vi "Autonomous Independent.vi"() -> ()   [LabVIEW 2016]
doc: "This VI is called when autonomous begins, and will automatically be terminated when autonomous ends. You can carry out timed or sensor driven robot movement independently without needing to return to the caller."
uses:
  <vilib>/Rock Robotics/WPI/Solenoid/WPI_SolenoidValue.ctl
  <vilib>/Rock Robotics/WPI/Utilities/WPI_GetSetVariantRefNum.vi
  <vilib>/Rock Robotics/Network Tables/NT Write Numeric Array.vi
  <vilib>/Rock Robotics/Network Tables/NT Read String.vi
  <vilib>/Rock Robotics/WPI/Solenoid/WPI_SolenoidSetEnum.vi
  Robot Global Data.vi
  <vilib>/Rock Robotics/Network Tables/NT Read Number.vi
panel:
  out "center x 8":dbl
  out "center y 8":dbl
  out "turn speed 7":dbl
  out "left motor 7":dbl
  out "right motor 7":dbl
  out "center x 7":dbl
  out "center y 7":dbl
  out "turn speed 6":dbl
  out "left motor 6":dbl
  out "right motor 6":dbl
  out "center x 6":dbl
  out "center y 6":dbl
  out "turn speed 5":dbl
  out "left motor 5":dbl
  out "right motor 5":dbl
  out "center x 2":dbl
  out "center y 2":dbl
  out "turn speed":dbl
  in  "turn offset":dbl
  out "left motor":dbl
  out "right motor":dbl
  in  "turn gain":dbl
  in  "drive gain":dbl
  in  "max drive speed":dbl
  in  "min drive speed":dbl
  in  "stop distance":dbl
  out "center x":dbl
  out "center y":dbl
  out "motor speed":dbl
  in  "setpoint":dbl
  # "Be sure to right-click and choose Data Operations>>Make Current Value default if you want to save the array values with the VI"
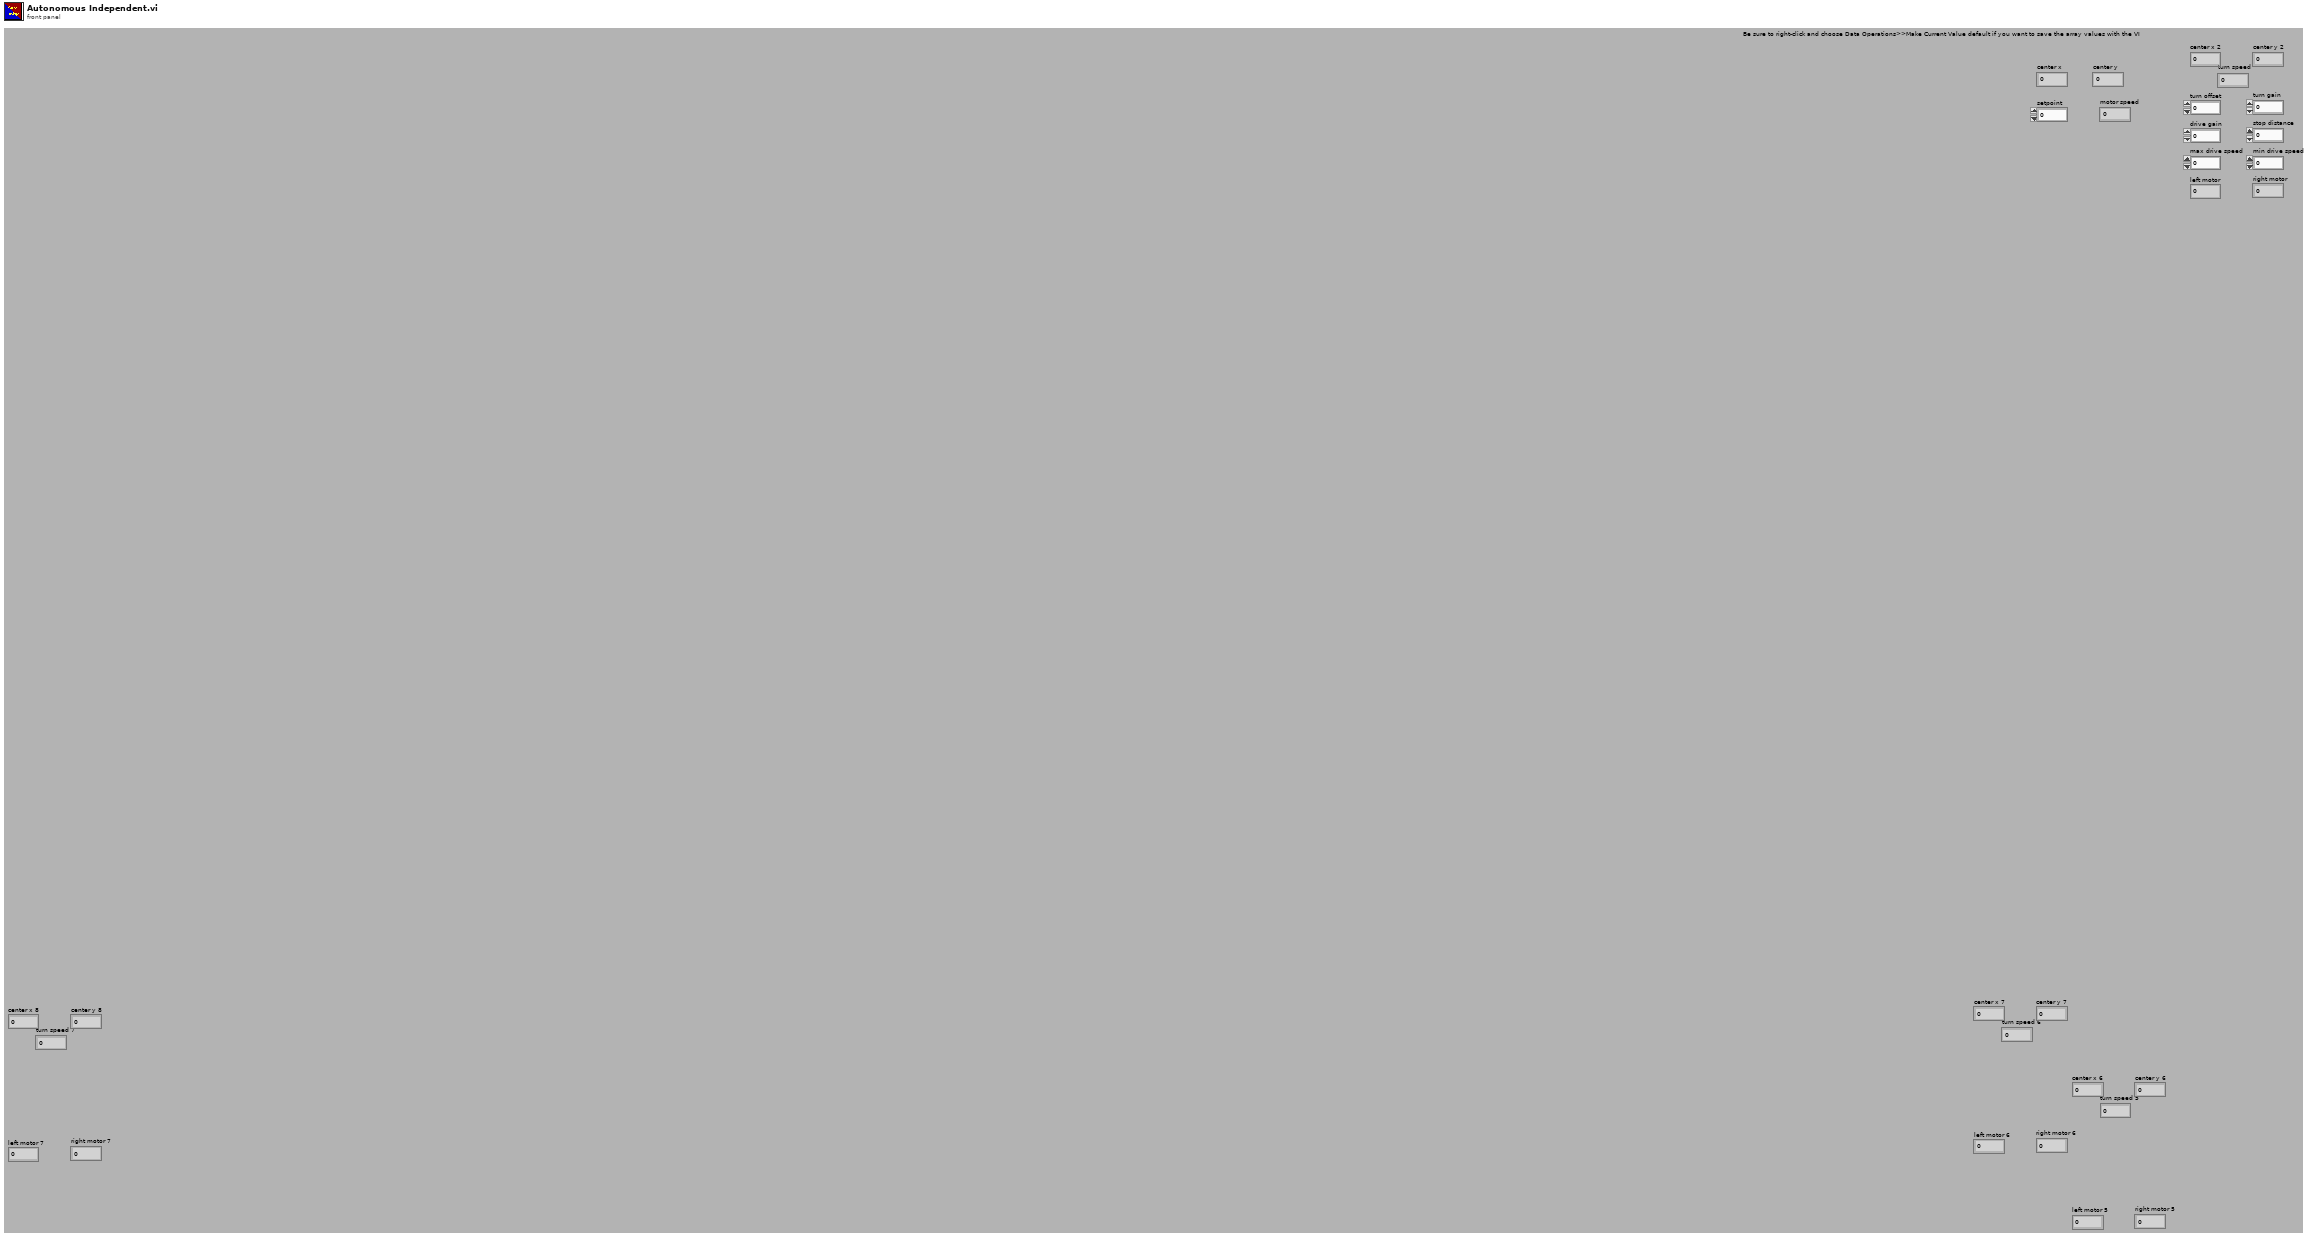
[diagram p1: front panel]
types:
  T1 = cluster{"Distance (ft)":dbl, "Score":dbl, "Normalized":cluster{"Center":cluster{dbl, dbl}, "Rectangle":cluster{"Numeric":dbl, "Numeric 2":dbl, "Numeric 3":dbl, "Numeric 5":dbl}}, "Pixels":cluster{"Center":cluster{dbl, dbl}, "Rectangle":cluster{"Numeric":dbl, "Numeric 2":dbl, "Numeric 3":dbl, "Numeric 5":dbl}}}
  T2 = typedef "WPI_RobotDriveDevRef.ctl" = cluster{"DevStatus":errorcluster, "Motors[]":T3[], "Square Inputs":bool, "Max Output":dbl}
  T3 = typedef "WPI_MotorControlDeviceRef.ctl" = cluster{"DeviceStatus":errorcluster, "Type":T4, "PWM":cluster{"PWM Channel":T5, "DeadBand":T6}, "CAN":cluster{"Device Number":u8, "SetOutput VI Ref":variant, "GetOutput VI Ref":variant, "Enable VI Ref":variant, "Disable VI Ref":variant, "Data":variant}, "Invert":bool}
  T4 = typedef "WPI_MotorControlType.ctl" = enum16{"PWM", "CAN"}
  T5 = typedef "FPGA_DIOPWMChannel.ctl" = enum8{"PWM 0", "PWM 1", "PWM 2", "PWM 3", "PWM 4", "PWM 5", "PWM 6", "PWM 7", "PWM 8", "PWM 9", "PWM MXP 0", "PWM MXP 1", "PWM MXP 2", "PWM MXP 3", "PWM MXP 4", "PWM MXP 5", "PWM MXP 6", "PWM MXP 7", "PWM MXP 8", "PWM MXP 9", "Invalid"}
  T6 = typedef "WPI_PWMDeadband.ctl" = cluster{"Name":string, "maxPositivePwm":i32, "minPositivePwm":i32, "centerPwm":i32, "maxNegativePwm":i32, "minNegativePwm":i32, "angularRange":u16}
  T7 = typedef "WPI_JoystickDevRef.ctl" = cluster{"Device":T8}
  T8 = typedef "WPI_JoystickDeviceEnum.ctl" = enum16{"USB 0", "USB 1", "USB 2", "USB 3", "USB 4", "USB 5"}
  T9 = typedef "WPI_SolenoidValue.ctl" = enum16{"Off", "On", "Forward", "Reverse"}
  T10 = typedef "WPI_EncoderDevRef.ctl" = cluster{"DevStatus":errorcluster, "EncoderIndex":T11, "CounterIndex":T12, "DistancePerCount":dbl, "Decoding Type":T13}
  T11 = typedef "FPGA_EncoderIdx.ctl" = enum8{"Enc 0", "Enc 1", "Enc 2", "Enc 3", "Enc 4", "Enc 5", "Enc 6", "Enc 7", "Invalid"}
  T12 = typedef "FPGA_CounterCtrSystemIndex.ctl" = enum8{"Ctr 0", "Ctr 1", "Ctr 2", "Ctr 3", "Ctr 4", "Ctr 5", "Ctr 6", "Ctr 7", "Invalid"}
  T13 = typedef "WPI_EncoderType.ctl" = enum16{"1x", "2x", "4x"}
  T14 = typedef "WPI_SolenoidDevRef.ctl" = cluster{"DevStatus":errorcluster, "Pneumatics Control Module":u8, "Forward Solenoid Channel":T15, "Reverse Solenoid Channel":T15}
  T15 = typedef "WPI_SolenoidChannel.ctl" = enum8{"Solenoid 0", "Solenoid 1", "Solenoid 2", "Solenoid 3", "Solenoid 4", "Solenoid 5", "Solenoid 6", "Solenoid 7", "Invalid"}
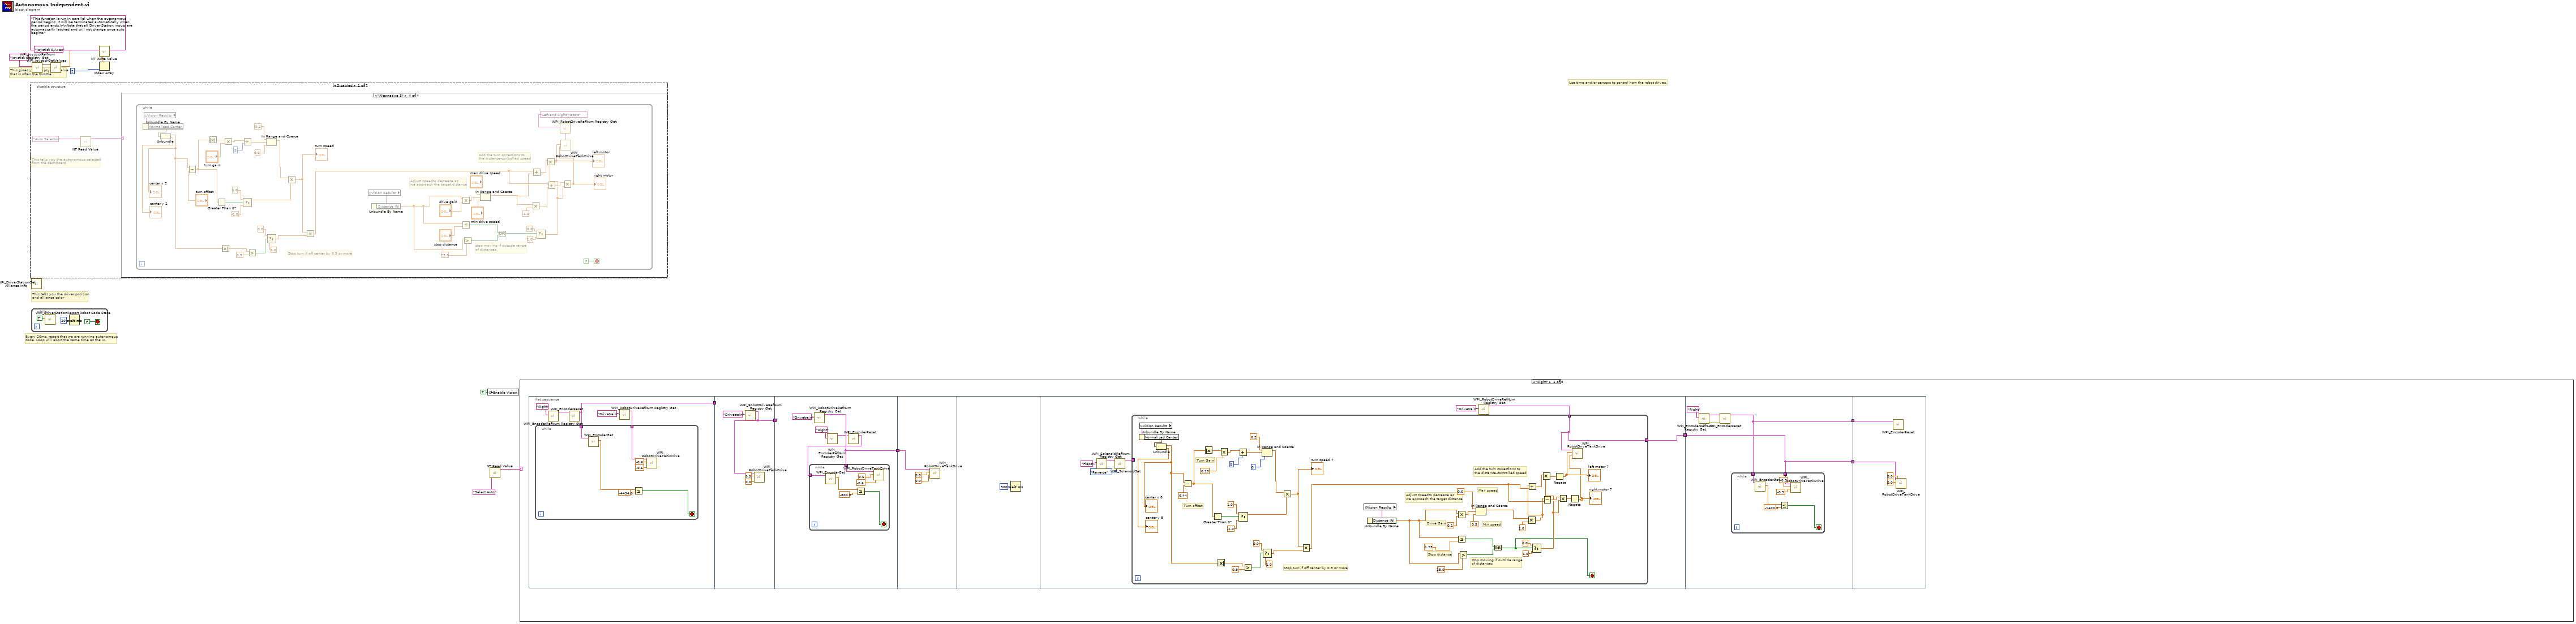
[diagram p0: block diagram]
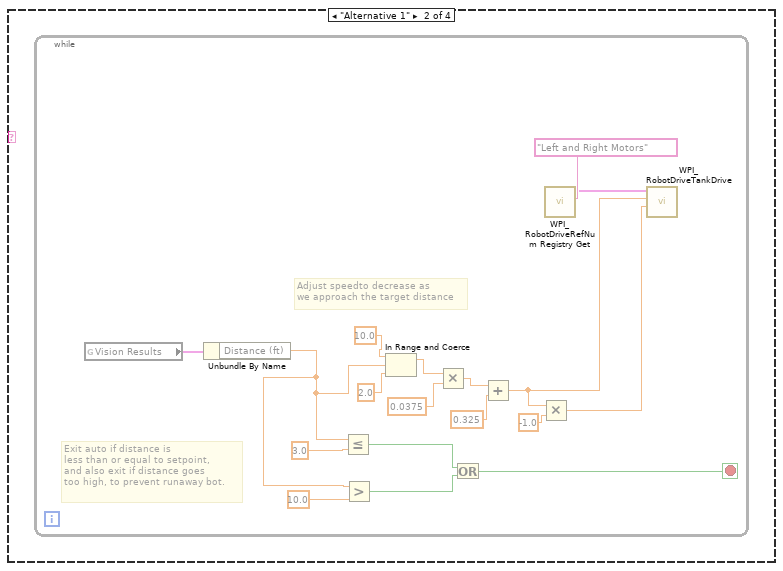
[diagram p3: hidden frame]
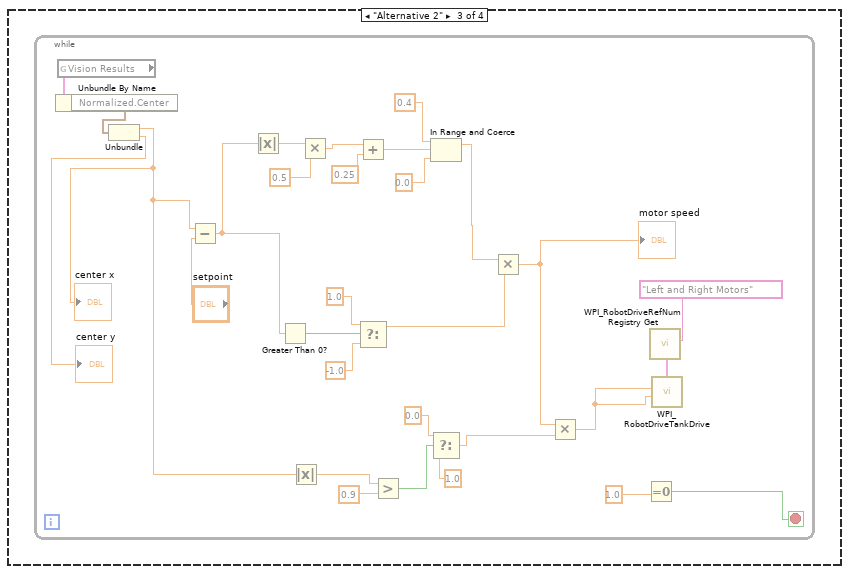
[diagram p4: hidden frame]
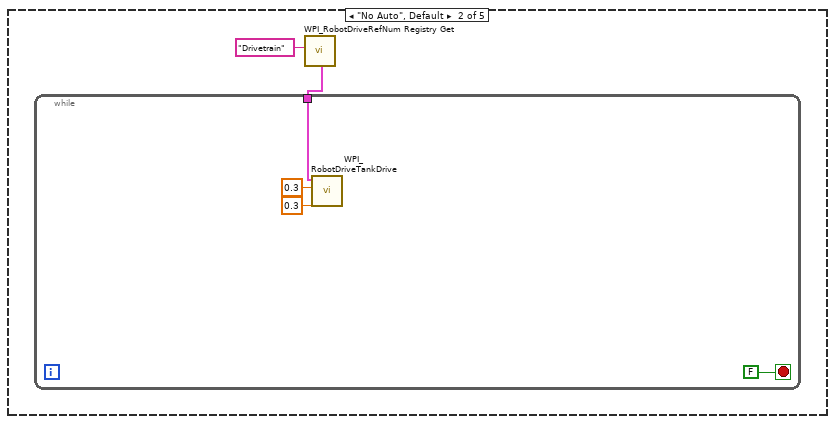
[diagram p6: hidden frame]
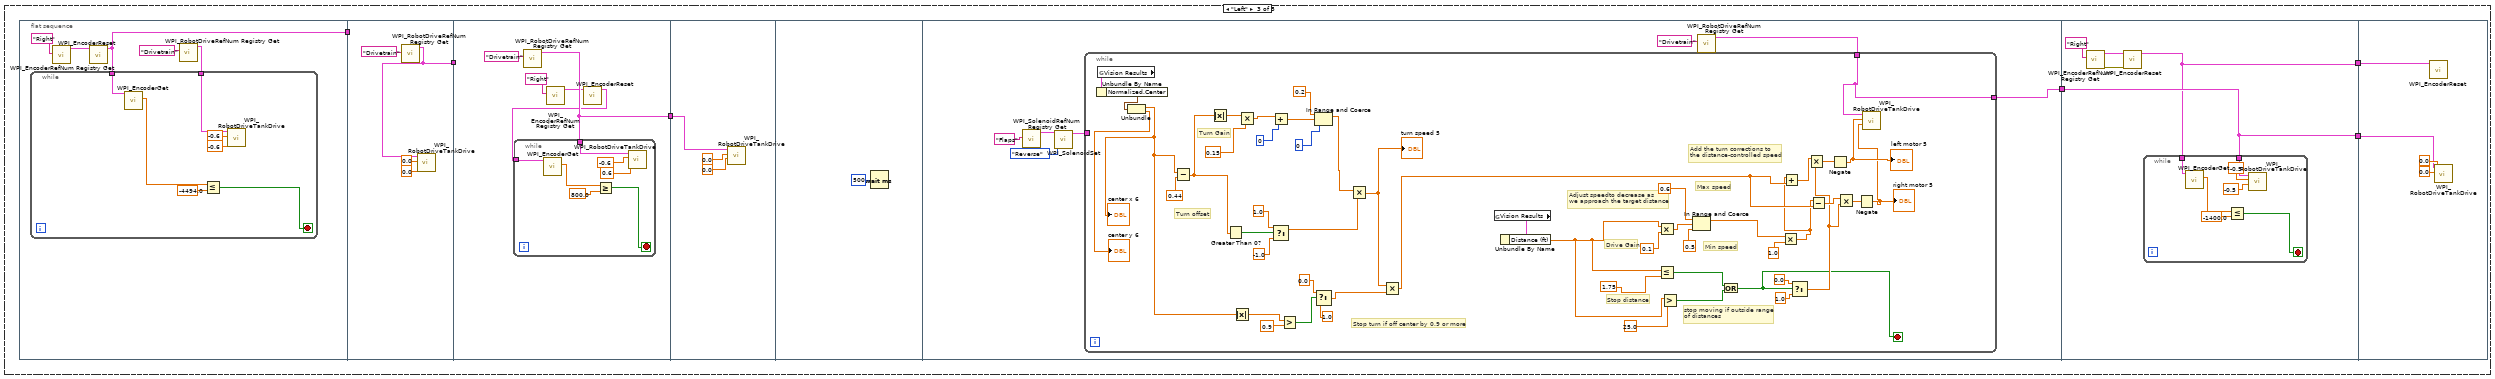
[diagram p7: hidden frame]
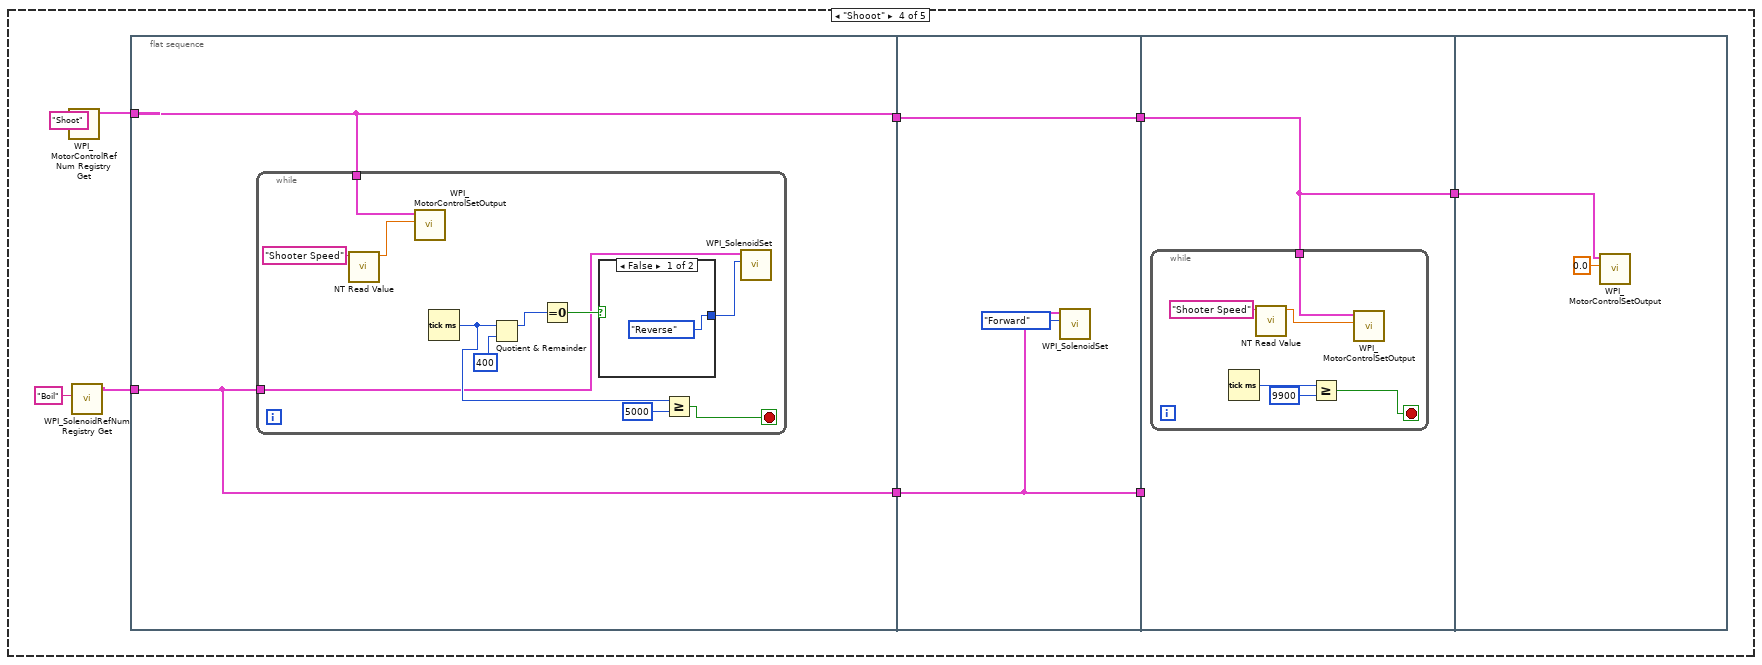
[diagram p8: hidden frame]
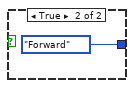
[diagram p9: hidden frame]
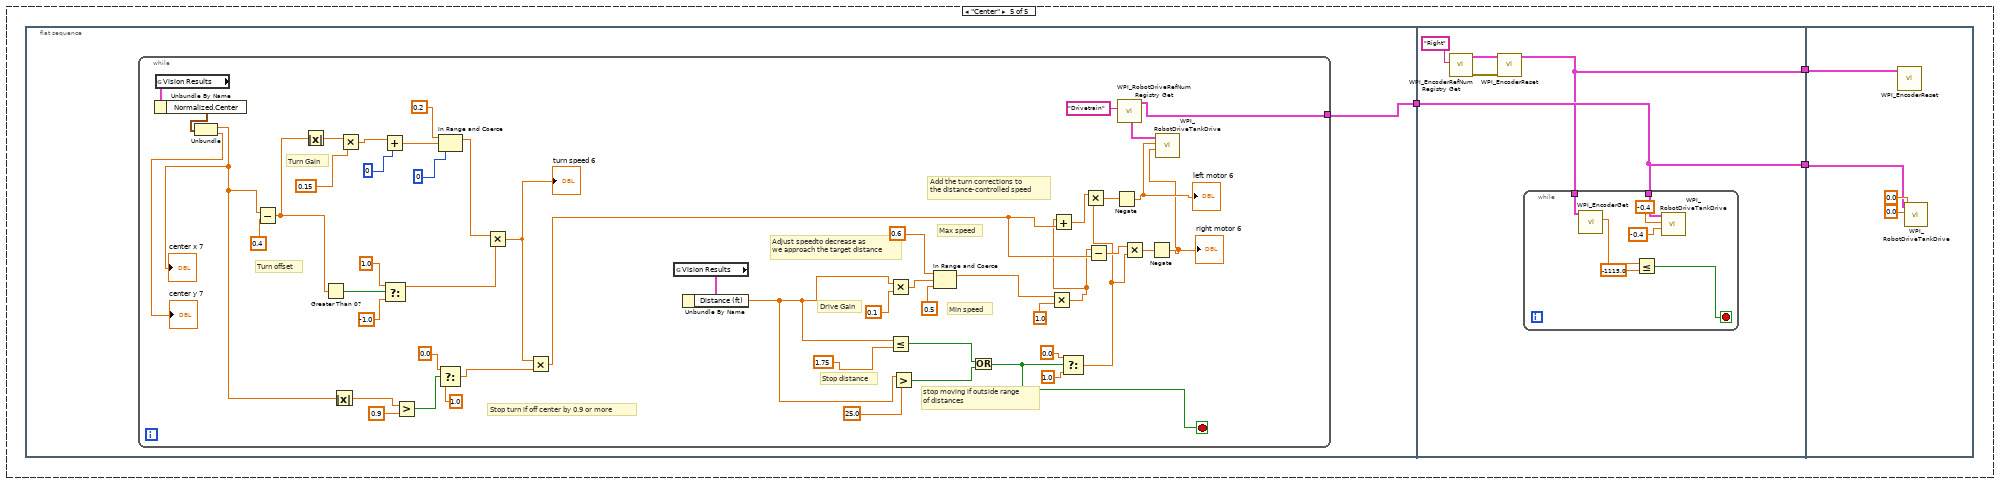
[diagram p10: hidden frame]
diagram:
  (unwired) "This function is run in parallel when the autonomous period begins. It will be terminated automatically when the period ends.\n\nNote that all Driver Station inputs are automatically latched and will not change once auto begins."
  # "Every 20ms, report that we are running autonomous\ncode. Loop will abort the same time as the VI."
  # "This gives you the joystick value\nthat is often the throttle"
  # "Use time and/or sensors to control how the robot drives."
  # "This tells you the driver position\nand alliance color"
  n1 = disable-structure shown="Disabled" {
    frame Disabled {
      # "This tells you the autonomous selected\nfrom the dashboard"
      n2 = call-poly <vilib>:"NT Read Value.vi"("Name"="Auto Selector") -> ("String"=w9:string)  [unwired: 9 in, 1 out]
      n3 = case shown="\"Alternative 3\"" w9 {
        frame Default {
          # "You can put your main auto here, or you can right-click on the case and make any\nother frame be the default case."
          # "This is the frame that will execute if no selection is made, or if it is not recognized"
        }
        frame "Alternative 1" {
          n4 = while {
            stop <- w11 stop-if-true
            # "Adjust speedto decrease as \nwe approach the target distance"
            # "Exit auto if distance is\nless than or equal to setpoint,\nand also exit if distance goes \ntoo high, to prevent runaway bot."
            n5 = global read "Robot Global Data.vi" "Vision Results"() -> (w28:T1)
            n6 = Unbundle By Name(w28) -> ("Distance (ft)"=w15:dbl)
            n7 = Less Or Equal?(x=w15, y=3.0) -> (x <= y?=w13:bool)
            n8 = Greater?(x=w15, y=10.0) -> (0:w12:bool)
            n9 = In Range and Coerce(upper limit=10.0 ("y"), x=w15, lower limit=2.0 ("y")) -> (coerced(x)=w22:dbl)  [unwired: 1 out]
            n10 = Multiply(x=w22, y=0.0375) -> (x*y=w20:dbl)
            n11 = Or(x=w13, y=w12) -> (x .or. y?=w11:bool)
            n12 = Add(x=w20, y=0.325) -> (x+y=w18:dbl)
            n13 = Multiply(x=w18, y=-1.0) -> (x*y=w16:dbl)
            n14 = call <vilib>:"WPI_RobotDriveRefNum Registry Get.vi"("refnum name"="Left and Right Motors") -> ("RobotDriveDevRef"=w26:T2)  [unwired: 9 in, 1 out]
            n15 = call <vilib>:"WPI_RobotDriveTankDrive.vi"("Right axis value"=w16, "Left axis value"=w18, "RobotDriveDevRef"=w26) -> ()  [unwired: 6 in, 3 out]
          }
        }
        frame "Alternative 2" {
          n16 = while {
            stop <- w32 stop-if-true
            n17 = global read "Robot Global Data.vi" "Vision Results"() -> (w58:T1)
            n18 = Unbundle By Name(w58) -> ("Normalized.Center"=w54:cluster{dbl, dbl})
            n19 = Unbundle(w54) -> (w30:dbl, →"center y":dbl)
            "center x" <- w30
            n20 = Subtract(x=w30, y="setpoint") -> (x-y=w29:dbl)
            n21 = Absolute Value(x=w29) -> (abs(x)=w46:dbl)
            n22 = Greater Than 0?(x=w29) -> (x > 0?=w51:bool)
            n23 = Absolute Value(x=w30) -> (abs(x)=w53:dbl)
            n24 = Multiply(x=w46, y=0.5) -> (x*y=w44:dbl)
            n25 = Add(x=w44, y=0.25) -> (x+y=w42:dbl)
            n26 = Select(t=1.0, s=w51, f=-1.0 ("t")) -> (s? t:f=w48:dbl)
            n27 = Greater?(x=w53, y=0.9) -> (0:w39:bool)
            n28 = In Range and Coerce(upper limit=0.4, x=w42, lower limit=0.0) -> (coerced(x)=w40:dbl)  [unwired: 1 out]
            n29 = Select(t=0.0, s=w39, f=1.0 ("t")) -> (s? t:f=w36:dbl)
            n30 = Multiply(x=w40, y=w48) -> (x*y=w35:dbl)
            "motor speed" <- w35
            n31 = Multiply(x=w35, y=w36) -> (x*y=w34:dbl)
            n32 = Equal To 0?(x=1.0 ("t")) -> (x = 0?=w32:bool)
            n33 = call <vilib>:"WPI_RobotDriveRefNum Registry Get.vi"("refnum name"="Left and Right Motors") -> ("RobotDriveDevRef"=w55:T2)  [unwired: 9 in, 1 out]
            n34 = call <vilib>:"WPI_RobotDriveTankDrive.vi"("Right axis value"=w34, "Left axis value"=w34, "RobotDriveDevRef"=w55) -> ()  [unwired: 6 in, 3 out]
          }
        }
        frame "Alternative 3" {
          n35 = while {
            stop <- FALSE stop-if-true
            # "stop moving if outside range\nof distances"
            # "Stop turn if off center by 0.9 or more"
            # "Add the turn corrections to \nthe distance-controlled speed"
            # "Adjust speedto decrease as \nwe approach the target distance"
            n36 = global read "Robot Global Data.vi" "Vision Results"() -> (w108:T1)
            n37 = Unbundle By Name(w108) -> ("Normalized.Center"=w106:cluster{dbl, dbl})
            n38 = Unbundle(w106) -> (w86:dbl, →"center y 2":dbl)
            "center x 2" <- w86
            n39 = Subtract(x=w86, y="turn offset") -> (x-y=w85:dbl)
            n40 = Absolute Value(x=w85) -> (abs(x)=w98:dbl)
            n41 = Greater Than 0?(x=w85) -> (x > 0?=w103:bool)
            n42 = Absolute Value(x=w86) -> (abs(x)=w105:dbl)
            n43 = Multiply(x=w98, y="turn gain") -> (x*y=w97:dbl)
            n44 = Add(x=w97, y=0) -> (x+y=w95:dbl)
            n45 = Select(t=1.0, s=w103, f=-1.0 ("t")) -> (s? t:f=w100:dbl)
            n46 = Greater?(x=w105, y=0.9) -> (0:w92:bool)
            n47 = In Range and Coerce(upper limit=0.2, x=w95, lower limit=0.0) -> (coerced(x)=w93:dbl)  [unwired: 1 out]
            n48 = Select(t=0.0, s=w92, f=1.0 ("t")) -> (s? t:f=w89:dbl)
            n49 = Multiply(x=w93, y=w100) -> (x*y=w88:dbl)
            "turn speed" <- w88
            n50 = Multiply(x=w88, y=w89) -> (x*y=w77:dbl)
            n51 = global read "Robot Global Data.vi" "Vision Results"() -> (w84:T1)
            n52 = Unbundle By Name(w84) -> ("Distance (ft)"=w65:dbl)
            n53 = Multiply(x=w65, y="drive gain") -> (x*y=w64:dbl)
            n54 = Less Or Equal?(x=w65, y="stop distance") -> (x <= y?=w79:bool)
            n55 = Greater?(x=w65, y=25.0) -> (0:w78:bool)
            n56 = In Range and Coerce(upper limit="max drive speed", x=w64, lower limit="min drive speed") -> (coerced(x)=w61:dbl)  [unwired: 1 out]
            n57 = Or(x=w79, y=w78) -> (x .or. y?=w75:bool)
            n58 = Multiply(x=w61, y=-1.0) -> (x*y=w76:dbl)
            n59 = Add(x=w77, y=w61) -> (x+y=w72:dbl)
            n60 = Select(t=0.0, s=w75, f=1.0 ("t")) -> (s? t:f=w70:dbl)
            n61 = Multiply(x=w72, y=w70) -> (x*y=w69:dbl)
            "left motor" <- w69
            n62 = Add(x=w77, y=w76) -> (x+y=w71:dbl)
            n63 = call <vilib>:"WPI_RobotDriveRefNum Registry Get.vi"("refnum name"="Left and Right Motors") -> ("RobotDriveDevRef"=w82:T2)  [unwired: 9 in, 1 out]
            n64 = Multiply(x=w71, y=w70) -> (x*y=w68:dbl)
            "right motor" <- w68
            n65 = call <vilib>:"WPI_RobotDriveTankDrive.vi"("Right axis value"=w68, "Left axis value"=w69, "RobotDriveDevRef"=w82) -> ()  [unwired: 6 in, 3 out]
          }
        }
      }
    }
    frame Enabled {
    }
  }
  n66 = while {
    stop <- FALSE stop-if-true
    n67 = call <vilib>:"WPI_DriverStationReport Robot Code State.vi"("Autonomous"=TRUE) -> ()  [unwired: 10 in, 1 out]
    n68 = Wait (ms)(milliseconds to wait=u32 20) -> ()  [unwired: 1 out]
  }
  n69 = call <vilib>:"WPI_DriverStationGet Alliance Info.vi"() -> ()  [unwired: 12 out]
  n70 = call <vilib>:"WPI_JoystickRefNum Registry Get.vi"("refnum name"="Joystick 0") -> ("JoystickDevRef"=w7:T7)  [unwired: 1 in, 9 out]
  n71 = call <vilib>:"WPI_JoystickGetValues.vi"("JoystickDevRef"=w7) -> ("Axes"=w5:dbl[])  [unwired: 6 in, 4 out]
  n72 = call-poly <vilib>:"NT Write Value.vi"("Numeric Array"=w5, "Name"="Joystick 0/Axes") -> ()  [unwired: 9 in, 1 out]
  n73 = Index Array(array=w5, index=2) -> ()  [unwired: 1 out]
  n74 = global write "Robot Global Data.vi" "Enable Vision"(TRUE ("Enable Vision")) -> ()
  n75 = call-poly <vilib>:"NT Read Value.vi"("Name"="Select Auto") -> ("String"=w2:string)  [unwired: 9 in, 1 out]
  n76 = case shown="\"Right\"" w2 {
    frame "Right" {
      n77 = flat-sequence {
        tunnel: [w118] -> w117
        tunnel: [w130] -> w116
        tunnel: w117 -> [_]
        tunnel: w116 -> [_]
        tunnel: [w137] -> w115
        tunnel: w115 -> [w146]
        tunnel: [w156] -> w114
        tunnel: w114 -> [w208]
        tunnel: [w208] -> w113
        tunnel: [w207] -> w112
        tunnel: w113 -> [w220]
        tunnel: w112 -> [w219]
        frame #0 {
          n78 = call <vilib>:"WPI_EncoderRefNum Registry Get.vi"("refnum name"="Right") -> ("EncoderDevRef"=w122:T10)  [unwired: 9 in, 1 out]
          n79 = call <vilib>:"WPI_EncoderReset.vi"("EncoderDevRef"=w122) -> ("EncoderDevRef"=w118:T10)  [unwired: 9 in, 1 out]
          n80 = call <vilib>:"WPI_RobotDriveRefNum Registry Get.vi"("refnum name"="Drivetrain") -> ("RobotDriveDevRef"=w119:T2)  [unwired: 9 in, 1 out]
          n81 = while {
            tunnel: w118 -> [w126]
            tunnel: w119 -> [w125]
            stop <- w127 stop-if-true
            n82 = call <vilib>:"WPI_EncoderGet.vi"("EncoderDevRef"=w126) -> ("Distance"=w129:dbl)  [unwired: 5 in, 5 out]
            n83 = Less Or Equal?(x=w129, y=-4494.0) -> (x <= y?=w127:bool)
            n84 = call <vilib>:"WPI_RobotDriveTankDrive.vi"("Right axis value"=-0.6, "Left axis value"=-0.6, "RobotDriveDevRef"=w125) -> ()  [unwired: 6 in, 3 out]
          }
        }
        frame #1 {
          n85 = call <vilib>:"WPI_RobotDriveRefNum Registry Get.vi"("refnum name"="Drivetrain") -> ("RobotDriveDevRef"=w130:T2)  [unwired: 9 in, 1 out]
          n86 = call <vilib>:"WPI_RobotDriveTankDrive.vi"("Right axis value"=0.0, "Left axis value"=0.0, "RobotDriveDevRef"=w130) -> ()  [unwired: 6 in, 3 out]
        }
        frame #2 {
          n87 = call <vilib>:"WPI_RobotDriveRefNum Registry Get.vi"("refnum name"="Drivetrain") -> ("RobotDriveDevRef"=w137:T2)  [unwired: 9 in, 1 out]
          n88 = call <vilib>:"WPI_EncoderRefNum Registry Get.vi"("refnum name"="Right") -> ("EncoderDevRef"=w136:T10)  [unwired: 9 in, 1 out]
          n89 = call <vilib>:"WPI_EncoderReset.vi"("EncoderDevRef"=w136) -> ("EncoderDevRef"=w134:T10)  [unwired: 9 in, 1 out]
          n90 = while {
            tunnel: w137 -> [w142]
            tunnel: w134 -> [w141]
            stop <- w145 stop-if-true
            n91 = call <vilib>:"WPI_EncoderGet.vi"("EncoderDevRef"=w141) -> ("Distance"=w140:dbl)  [unwired: 5 in, 5 out]
            n92 = Less Or Equal?(x=w140, y=-800.0) -> (x <= y?=w145:bool)
            n93 = call <vilib>:"WPI_RobotDriveTankDrive.vi"("Right axis value"=-0.6, "Left axis value"=0.6, "RobotDriveDevRef"=w142) -> ()  [unwired: 6 in, 3 out]
          }
        }
        frame #3 {
          n94 = call <vilib>:"WPI_RobotDriveTankDrive.vi"("Right axis value"=0.0, "Left axis value"=0.0, "RobotDriveDevRef"=w146) -> ()  [unwired: 6 in, 3 out]
        }
        frame #4 {
          n95 = Wait (ms)(milliseconds to wait=u32 500) -> ()  [unwired: 1 out]
        }
        frame #5 {
          n96 = call <vilib>:"WPI_SolenoidRefNum Registry Get.vi"("refnum name"="Flaps") -> ("SolenoidDevRef"=w154:T14)  [unwired: 9 in, 1 out]
          n97 = call-poly <vilib>:"WPI_SolenoidSet.vi"("Value"=WPI_SolenoidValue."Reverse", "SolenoidDevRef"=w154) -> ("SolenoidDevRef"=w150:T14)  [unwired: 8 in, 1 out]
          n98 = call <vilib>:"WPI_RobotDriveRefNum Registry Get.vi"("refnum name"="Drivetrain") -> ("RobotDriveDevRef"=w151:T2)  [unwired: 9 in, 1 out]
          n99 = while {
            tunnel: [w158] -> w156
            tunnel: w151 -> [w158]
            tunnel: w150 -> [_]
            stop <- w157 stop-if-true
            # "Min speed"
            # "Max speed"
            # "Stop distance"
            # "Drive Gain"
            # "Turn offset"
            # "Turn Gain"
            # "stop moving if outside range\nof distances"
            # "Stop turn if off center by 0.9 or more"
            # "Add the turn corrections to \nthe distance-controlled speed"
            # "Adjust speedto decrease as \nwe approach the target distance"
            n100 = global read "Robot Global Data.vi" "Vision Results"() -> (w206:T1)
            n101 = Unbundle By Name(w206) -> ("Normalized.Center"=w204:cluster{dbl, dbl})
            n102 = Unbundle(w204) -> (w185:dbl, →"center y 8":dbl)
            "center x 8" <- w185
            n103 = Subtract(x=w185, y=0.44) -> (x-y=w184:dbl)
            n104 = Absolute Value(x=w184) -> (abs(x)=w196:dbl)
            n105 = Greater Than 0?(x=w184) -> (x > 0?=w201:bool)
            n106 = Absolute Value(x=w185) -> (abs(x)=w203:dbl)
            n107 = Multiply(x=w196, y=0.15) -> (x*y=w195:dbl)
            n108 = Add(x=w195, y=0) -> (x+y=w193:dbl)
            n109 = Select(t=1.0, s=w201, f=-1.0 ("t")) -> (s? t:f=w198:dbl)
            n110 = Greater?(x=w203, y=0.9) -> (0:w190:bool)
            n111 = In Range and Coerce(upper limit=0.2, x=w193, lower limit=0) -> (coerced(x)=w191:dbl)  [unwired: 1 out]
            n112 = Select(t=0.0, s=w190, f=1.0 ("t")) -> (s? t:f=w187:dbl)
            n113 = Multiply(x=w191, y=w198) -> (x*y=w186:dbl)
            "turn speed 7" <- w186
            n114 = Multiply(x=w186, y=w187) -> (x*y=w164:dbl)
            n115 = global read "Robot Global Data.vi" "Vision Results"() -> (w183:T1)
            n116 = Unbundle By Name(w183) -> ("Distance (ft)"=w173:dbl)
            n117 = Multiply(x=w173, y=0.1) -> (x*y=w172:dbl)
            n118 = Less Or Equal?(x=w173, y=1.75) -> (x <= y?=w180:bool)
            n119 = Greater?(x=w173, y=25.0) -> (0:w179:bool)
            n120 = In Range and Coerce(upper limit=0.6, x=w172, lower limit=0.5) -> (coerced(x)=w171:dbl)  [unwired: 1 out]
            n121 = Or(x=w180, y=w179) -> (x .or. y?=w157:bool)
            n122 = Multiply(x=w171, y=1.0) -> (x*y=w163:dbl)
            n123 = Add(x=w163, y=w164) -> (x+y=w176:dbl)
            n124 = Select(t=0.0, s=w157, f=1.0 ("t")) -> (s? t:f=w174:dbl)
            n125 = Multiply(x=w176, y=w174) -> (x*y=w162:dbl)
            n126 = Subtract(x=w163, y=w164) -> (x-y=w175:dbl)
            n127 = Negate(x=w162) -> (-x=w161:dbl)
            "left motor 7" <- w161
            n128 = Multiply(x=w175, y=w174) -> (x*y=w160:dbl)
            n129 = Negate(x=w160) -> (-x=w159:dbl)
            "right motor 7" <- w159
            n130 = call <vilib>:"WPI_RobotDriveTankDrive.vi"("Right axis value"=w159, "Left axis value"=w161, "RobotDriveDevRef"=w158) -> ()  [unwired: 6 in, 3 out]
          }
        }
        frame #6 {
          n131 = call <vilib>:"WPI_EncoderRefNum Registry Get.vi"("refnum name"="Right") -> ("error out"=w210:errorcluster, "EncoderDevRef"=w209:T10)  [unwired: 9 in]
          n132 = call <vilib>:"WPI_EncoderReset.vi"("error in (no error)"=w210, "EncoderDevRef"=w209) -> ("EncoderDevRef"=w207:T10)  [unwired: 8 in, 1 out]
          n133 = while {
            tunnel: w207 -> [w218]
            tunnel: w208 -> [w214]
            stop <- w215 stop-if-true
            n134 = call <vilib>:"WPI_EncoderGet.vi"("EncoderDevRef"=w218) -> ("Distance"=w217:dbl)  [unwired: 5 in, 5 out]
            n135 = Less Or Equal?(x=w217, y=-1400.0) -> (x <= y?=w215:bool)
            n136 = call <vilib>:"WPI_RobotDriveTankDrive.vi"("Right axis value"=-0.5 ("Left axis value"), "Left axis value"=-0.5 ("Right axis value"), "RobotDriveDevRef"=w214) -> ()  [unwired: 6 in, 3 out]
          }
        }
        frame #7 {
          n137 = call <vilib>:"WPI_EncoderReset.vi"("EncoderDevRef"=w219) -> ()  [unwired: 9 in, 2 out]
          n138 = call <vilib>:"WPI_RobotDriveTankDrive.vi"("Right axis value"=0.0, "Left axis value"=0.0, "RobotDriveDevRef"=w220) -> ()  [unwired: 6 in, 3 out]
        }
      }
    }
    frame "No Auto", Default {
      n139 = call <vilib>:"WPI_RobotDriveRefNum Registry Get.vi"("refnum name"="Drivetrain") -> ("RobotDriveDevRef"=w223:T2)  [unwired: 9 in, 1 out]
      n140 = while {
        tunnel: w223 -> [w225]
        stop <- FALSE stop-if-true
        n141 = call <vilib>:"WPI_RobotDriveTankDrive.vi"("Right axis value"=0.3, "Left axis value"=0.3, "RobotDriveDevRef"=w225) -> ()  [unwired: 6 in, 3 out]
      }
    }
    frame "Left" {
      n142 = flat-sequence {
        tunnel: [w235] -> w229
        tunnel: [w247] -> w230
        tunnel: w229 -> [_]
        tunnel: w230 -> [_]
        tunnel: [w254] -> w231
        tunnel: w231 -> [w263]
        tunnel: [w273] -> w234
        tunnel: w234 -> [w325]
        tunnel: [w325] -> w233
        tunnel: [w324] -> w232
        tunnel: w233 -> [w337]
        tunnel: w232 -> [w336]
        frame #0 {
          n143 = call <vilib>:"WPI_EncoderRefNum Registry Get.vi"("refnum name"="Right") -> ("EncoderDevRef"=w239:T10)  [unwired: 9 in, 1 out]
          n144 = call <vilib>:"WPI_EncoderReset.vi"("EncoderDevRef"=w239) -> ("EncoderDevRef"=w235:T10)  [unwired: 9 in, 1 out]
          n145 = call <vilib>:"WPI_RobotDriveRefNum Registry Get.vi"("refnum name"="Drivetrain") -> ("RobotDriveDevRef"=w236:T2)  [unwired: 9 in, 1 out]
          n146 = while {
            tunnel: w235 -> [w243]
            tunnel: w236 -> [w242]
            stop <- w244 stop-if-true
            n147 = call <vilib>:"WPI_EncoderGet.vi"("EncoderDevRef"=w243) -> ("Distance"=w246:dbl)  [unwired: 5 in, 5 out]
            n148 = Less Or Equal?(x=w246, y=-4494.0) -> (x <= y?=w244:bool)
            n149 = call <vilib>:"WPI_RobotDriveTankDrive.vi"("Right axis value"=-0.6, "Left axis value"=-0.6, "RobotDriveDevRef"=w242) -> ()  [unwired: 6 in, 3 out]
          }
        }
        frame #1 {
          n150 = call <vilib>:"WPI_RobotDriveRefNum Registry Get.vi"("refnum name"="Drivetrain") -> ("RobotDriveDevRef"=w247:T2)  [unwired: 9 in, 1 out]
          n151 = call <vilib>:"WPI_RobotDriveTankDrive.vi"("Right axis value"=0.0, "Left axis value"=0.0, "RobotDriveDevRef"=w247) -> ()  [unwired: 6 in, 3 out]
        }
        frame #2 {
          n152 = call <vilib>:"WPI_RobotDriveRefNum Registry Get.vi"("refnum name"="Drivetrain") -> ("RobotDriveDevRef"=w254:T2)  [unwired: 9 in, 1 out]
          n153 = call <vilib>:"WPI_EncoderRefNum Registry Get.vi"("refnum name"="Right") -> ("EncoderDevRef"=w253:T10)  [unwired: 9 in, 1 out]
          n154 = call <vilib>:"WPI_EncoderReset.vi"("EncoderDevRef"=w253) -> ("EncoderDevRef"=w251:T10)  [unwired: 9 in, 1 out]
          n155 = while {
            tunnel: w254 -> [w259]
            tunnel: w251 -> [w258]
            stop <- w262 stop-if-true
            n156 = call <vilib>:"WPI_EncoderGet.vi"("EncoderDevRef"=w258) -> ("Distance"=w257:dbl)  [unwired: 5 in, 5 out]
            n157 = Greater Or Equal?(x=w257, y=800.0) -> (x >= y?=w262:bool)
            n158 = call <vilib>:"WPI_RobotDriveTankDrive.vi"("Right axis value"=0.6, "Left axis value"=-0.6, "RobotDriveDevRef"=w259) -> ()  [unwired: 6 in, 3 out]
          }
        }
        frame #3 {
          n159 = call <vilib>:"WPI_RobotDriveTankDrive.vi"("Right axis value"=0.0, "Left axis value"=0.0, "RobotDriveDevRef"=w263) -> ()  [unwired: 6 in, 3 out]
        }
        frame #4 {
          n160 = Wait (ms)(milliseconds to wait=u32 500) -> ()  [unwired: 1 out]
        }
        frame #5 {
          n161 = call <vilib>:"WPI_SolenoidRefNum Registry Get.vi"("refnum name"="Flaps") -> ("SolenoidDevRef"=w271:T14)  [unwired: 9 in, 1 out]
          n162 = call-poly <vilib>:"WPI_SolenoidSet.vi"("Value"=WPI_SolenoidValue."Reverse", "SolenoidDevRef"=w271) -> ("SolenoidDevRef"=w267:T14)  [unwired: 8 in, 1 out]
          n163 = call <vilib>:"WPI_RobotDriveRefNum Registry Get.vi"("refnum name"="Drivetrain") -> ("RobotDriveDevRef"=w268:T2)  [unwired: 9 in, 1 out]
          n164 = while {
            tunnel: [w275] -> w273
            tunnel: w268 -> [w275]
            tunnel: w267 -> [_]
            stop <- w274 stop-if-true
            # "Min speed"
            # "Max speed"
            # "Stop distance"
            # "Drive Gain"
            # "Turn offset"
            # "Turn Gain"
            # "stop moving if outside range\nof distances"
            # "Stop turn if off center by 0.9 or more"
            # "Add the turn corrections to \nthe distance-controlled speed"
            # "Adjust speedto decrease as \nwe approach the target distance"
            n165 = global read "Robot Global Data.vi" "Vision Results"() -> (w323:T1)
            n166 = Unbundle By Name(w323) -> ("Normalized.Center"=w321:cluster{dbl, dbl})
            n167 = Unbundle(w321) -> (w302:dbl, →"center y 6":dbl)
            "center x 6" <- w302
            n168 = Subtract(x=w302, y=0.44) -> (x-y=w301:dbl)
            n169 = Absolute Value(x=w301) -> (abs(x)=w313:dbl)
            n170 = Greater Than 0?(x=w301) -> (x > 0?=w318:bool)
            n171 = Absolute Value(x=w302) -> (abs(x)=w320:dbl)
            n172 = Multiply(x=w313, y=0.15) -> (x*y=w312:dbl)
            n173 = Add(x=w312, y=0) -> (x+y=w310:dbl)
            n174 = Select(t=1.0, s=w318, f=-1.0 ("t")) -> (s? t:f=w315:dbl)
            n175 = Greater?(x=w320, y=0.9) -> (0:w307:bool)
            n176 = In Range and Coerce(upper limit=0.2, x=w310, lower limit=0) -> (coerced(x)=w308:dbl)  [unwired: 1 out]
            n177 = Select(t=0.0, s=w307, f=1.0 ("t")) -> (s? t:f=w304:dbl)
            n178 = Multiply(x=w308, y=w315) -> (x*y=w303:dbl)
            "turn speed 5" <- w303
            n179 = Multiply(x=w303, y=w304) -> (x*y=w281:dbl)
            n180 = global read "Robot Global Data.vi" "Vision Results"() -> (w300:T1)
            n181 = Unbundle By Name(w300) -> ("Distance (ft)"=w290:dbl)
            n182 = Multiply(x=w290, y=0.1) -> (x*y=w289:dbl)
            n183 = Less Or Equal?(x=w290, y=1.75) -> (x <= y?=w297:bool)
            n184 = Greater?(x=w290, y=25.0) -> (0:w296:bool)
            n185 = In Range and Coerce(upper limit=0.6, x=w289, lower limit=0.5) -> (coerced(x)=w288:dbl)  [unwired: 1 out]
            n186 = Or(x=w297, y=w296) -> (x .or. y?=w274:bool)
            n187 = Multiply(x=w288, y=1.0) -> (x*y=w280:dbl)
            n188 = Add(x=w280, y=w281) -> (x+y=w293:dbl)
            n189 = Select(t=0.0, s=w274, f=1.0 ("t")) -> (s? t:f=w291:dbl)
            n190 = Multiply(x=w293, y=w291) -> (x*y=w279:dbl)
            n191 = Subtract(x=w280, y=w281) -> (x-y=w292:dbl)
            n192 = Negate(x=w279) -> (-x=w278:dbl)
            "left motor 5" <- w278
            n193 = Multiply(x=w292, y=w291) -> (x*y=w277:dbl)
            n194 = Negate(x=w277) -> (-x=w276:dbl)
            "right motor 5" <- w276
            n195 = call <vilib>:"WPI_RobotDriveTankDrive.vi"("Right axis value"=w276, "Left axis value"=w278, "RobotDriveDevRef"=w275) -> ()  [unwired: 6 in, 3 out]
          }
        }
        frame #6 {
          n196 = call <vilib>:"WPI_EncoderRefNum Registry Get.vi"("refnum name"="Right") -> ("error out"=w327:errorcluster, "EncoderDevRef"=w326:T10)  [unwired: 9 in]
          n197 = call <vilib>:"WPI_EncoderReset.vi"("error in (no error)"=w327, "EncoderDevRef"=w326) -> ("EncoderDevRef"=w324:T10)  [unwired: 8 in, 1 out]
          n198 = while {
            tunnel: w324 -> [w335]
            tunnel: w325 -> [w331]
            stop <- w332 stop-if-true
            n199 = call <vilib>:"WPI_EncoderGet.vi"("EncoderDevRef"=w335) -> ("Distance"=w334:dbl)  [unwired: 5 in, 5 out]
            n200 = Less Or Equal?(x=w334, y=-1400.0) -> (x <= y?=w332:bool)
            n201 = call <vilib>:"WPI_RobotDriveTankDrive.vi"("Right axis value"=-0.5 ("Left axis value"), "Left axis value"=-0.5 ("Right axis value"), "RobotDriveDevRef"=w331) -> ()  [unwired: 6 in, 3 out]
          }
        }
        frame #7 {
          n202 = call <vilib>:"WPI_EncoderReset.vi"("EncoderDevRef"=w336) -> ()  [unwired: 9 in, 2 out]
          n203 = call <vilib>:"WPI_RobotDriveTankDrive.vi"("Right axis value"=0.0, "Left axis value"=0.0, "RobotDriveDevRef"=w337) -> ()  [unwired: 6 in, 3 out]
        }
      }
    }
    frame "Shooot" {
      n204 = call <vilib>:"WPI_MotorControlRefNum Registry Get.vi"("refnum name"="Shoot") -> ("MotorControlDevRef"=w347:T3)  [unwired: 9 in, 1 out]
      n205 = call <vilib>:"WPI_SolenoidRefNum Registry Get.vi"("refnum name"="Boil") -> ("SolenoidDevRef"=w344:T14)  [unwired: 9 in, 1 out]
      n206 = flat-sequence {
        tunnel: w347 -> [w350]
        tunnel: [w350] -> w343
        tunnel: w344 -> [w349]
        tunnel: [w349] -> w341
        tunnel: w343 -> [w366]
        tunnel: [w366] -> w342
        tunnel: w341 -> [w365]
        tunnel: [w365] -> w340
        tunnel: w342 -> [w367]
        tunnel: [w367] -> w346
        tunnel: w340 -> [_]
        tunnel: w346 -> [w375]
        frame #0 {
          n207 = while {
            tunnel: w350 -> [w359]
            tunnel: w349 -> [w351]
            stop <- w352 stop-if-true
            n208 = call-poly <vilib>:"NT Read Value.vi"("Name"="Shooter Speed") -> ("Numeric"=w360:dbl)  [unwired: 9 in, 1 out]
            n209 = call <vilib>:"WPI_MotorControlSetOutput.vi"("Output"=w360, "MotorControlDevRef"=w359) -> ()  [unwired: 7 in, 3 out]
            n210 = Tick Count (ms)() -> (millisecond timer value=w354:u32)
            n211 = Quotient & Remainder(x=w354, y=u32 400) -> (x-y*floor(x/y)=w357:u32)  [unwired: 1 out]
            n212 = Equal To 0?(x=w357) -> (x = 0?=w356:bool)
            n213 = case shown="False" w356 {
              tunnel: [WPI_SolenoidValue."Reverse" ("Value") WPI_SolenoidValue."Forward" ("Value")] -> w355
              frame False {
              }
              frame True {
              }
            }
            n214 = Greater Or Equal?(x=w354, y=u32 5000) -> (x >= y?=w352:bool)
            n215 = call-poly <vilib>:"WPI_SolenoidSet.vi"("Value"=w355, "SolenoidDevRef"=w351) -> ()  [unwired: 8 in, 2 out]
          }
        }
        frame #1 {
          n216 = call-poly <vilib>:"WPI_SolenoidSet.vi"("Value"=WPI_SolenoidValue."Forward", "SolenoidDevRef"=w365) -> ()  [unwired: 8 in, 2 out]
        }
        frame #2 {
          n217 = while {
            tunnel: w367 -> [w371]
            stop <- w368 stop-if-true
            n218 = Tick Count (ms)() -> (millisecond timer value=w370:u32)
            n219 = call-poly <vilib>:"NT Read Value.vi"("Name"="Shooter Speed") -> ("Numeric"=w372:dbl)  [unwired: 9 in, 1 out]
            n220 = Greater Or Equal?(x=w370, y=u32 9900) -> (x >= y?=w368:bool)
            n221 = call <vilib>:"WPI_MotorControlSetOutput.vi"("Output"=w372, "MotorControlDevRef"=w371) -> ()  [unwired: 7 in, 3 out]
          }
        }
        frame #3 {
          n222 = call <vilib>:"WPI_MotorControlSetOutput.vi"("Output"=0.0, "MotorControlDevRef"=w375) -> ()  [unwired: 7 in, 3 out]
        }
      }
    }
    frame "Center" {
      n223 = flat-sequence {
        tunnel: [w379] -> w378
        tunnel: w378 -> [w432]
        tunnel: [w432] -> w377
        tunnel: [w431] -> w376
        tunnel: w377 -> [w444]
        tunnel: w376 -> [w443]
        frame #0 {
          n224 = while {
            tunnel: [w381] -> w379
            stop <- w380 stop-if-true
            # "Min speed"
            # "Max speed"
            # "Stop distance"
            # "Drive Gain"
            # "Turn offset"
            # "Turn Gain"
            # "stop moving if outside range\nof distances"
            # "Stop turn if off center by 0.9 or more"
            # "Add the turn corrections to \nthe distance-controlled speed"
            # "Adjust speedto decrease as \nwe approach the target distance"
            n225 = global read "Robot Global Data.vi" "Vision Results"() -> (w430:T1)
            n226 = Unbundle By Name(w430) -> ("Normalized.Center"=w428:cluster{dbl, dbl})
            n227 = Unbundle(w428) -> (w409:dbl, →"center y 7":dbl)
            "center x 7" <- w409
            n228 = Subtract(x=w409, y=0.4) -> (x-y=w408:dbl)
            n229 = Absolute Value(x=w408) -> (abs(x)=w420:dbl)
            n230 = Greater Than 0?(x=w408) -> (x > 0?=w425:bool)
            n231 = Absolute Value(x=w409) -> (abs(x)=w427:dbl)
            n232 = Multiply(x=w420, y=0.15) -> (x*y=w419:dbl)
            n233 = Add(x=w419, y=0) -> (x+y=w417:dbl)
            n234 = Select(t=1.0, s=w425, f=-1.0 ("t")) -> (s? t:f=w422:dbl)
            n235 = Greater?(x=w427, y=0.9) -> (0:w414:bool)
            n236 = In Range and Coerce(upper limit=0.2, x=w417, lower limit=0) -> (coerced(x)=w415:dbl)  [unwired: 1 out]
            n237 = Select(t=0.0, s=w414, f=1.0 ("t")) -> (s? t:f=w411:dbl)
            n238 = Multiply(x=w415, y=w422) -> (x*y=w410:dbl)
            "turn speed 6" <- w410
            n239 = Multiply(x=w410, y=w411) -> (x*y=w387:dbl)
            n240 = global read "Robot Global Data.vi" "Vision Results"() -> (w407:T1)
            n241 = Unbundle By Name(w407) -> ("Distance (ft)"=w397:dbl)
            n242 = Multiply(x=w397, y=0.1) -> (x*y=w396:dbl)
            n243 = Less Or Equal?(x=w397, y=1.75) -> (x <= y?=w404:bool)
            n244 = Greater?(x=w397, y=25.0) -> (0:w403:bool)
            n245 = In Range and Coerce(upper limit=0.6, x=w396, lower limit=0.5) -> (coerced(x)=w395:dbl)  [unwired: 1 out]
            n246 = Or(x=w404, y=w403) -> (x .or. y?=w380:bool)
            n247 = Multiply(x=w395, y=1.0) -> (x*y=w386:dbl)
            n248 = Add(x=w386, y=w387) -> (x+y=w400:dbl)
            n249 = Select(t=0.0, s=w380, f=1.0 ("t")) -> (s? t:f=w398:dbl)
            n250 = Multiply(x=w400, y=w398) -> (x*y=w385:dbl)
            n251 = Subtract(x=w386, y=w387) -> (x-y=w399:dbl)
            n252 = Negate(x=w385) -> (-x=w384:dbl)
            "left motor 6" <- w384
            n253 = call <vilib>:"WPI_RobotDriveRefNum Registry Get.vi"("refnum name"="Drivetrain") -> ("RobotDriveDevRef"=w381:T2)  [unwired: 9 in, 1 out]
            n254 = Multiply(x=w399, y=w398) -> (x*y=w383:dbl)
            n255 = Negate(x=w383) -> (-x=w382:dbl)
            "right motor 6" <- w382
            n256 = call <vilib>:"WPI_RobotDriveTankDrive.vi"("Right axis value"=w382, "Left axis value"=w384, "RobotDriveDevRef"=w381) -> ()  [unwired: 6 in, 3 out]
          }
        }
        frame #1 {
          n257 = call <vilib>:"WPI_EncoderRefNum Registry Get.vi"("refnum name"="Right") -> ("error out"=w434:errorcluster, "EncoderDevRef"=w433:T10)  [unwired: 9 in]
          n258 = call <vilib>:"WPI_EncoderReset.vi"("error in (no error)"=w434, "EncoderDevRef"=w433) -> ("EncoderDevRef"=w431:T10)  [unwired: 8 in, 1 out]
          n259 = while {
            tunnel: w431 -> [w442]
            tunnel: w432 -> [w438]
            stop <- w439 stop-if-true
            n260 = call <vilib>:"WPI_EncoderGet.vi"("EncoderDevRef"=w442) -> ("Distance"=w441:dbl)  [unwired: 5 in, 5 out]
            n261 = Less Or Equal?(x=w441, y=-1115.0) -> (x <= y?=w439:bool)
            n262 = call <vilib>:"WPI_RobotDriveTankDrive.vi"("Right axis value"=-0.4 ("Left axis value"), "Left axis value"=-0.4 ("Right axis value"), "RobotDriveDevRef"=w438) -> ()  [unwired: 6 in, 3 out]
          }
        }
        frame #2 {
          n263 = call <vilib>:"WPI_EncoderReset.vi"("EncoderDevRef"=w443) -> ()  [unwired: 9 in, 2 out]
          n264 = call <vilib>:"WPI_RobotDriveTankDrive.vi"("Right axis value"=0.0, "Left axis value"=0.0, "RobotDriveDevRef"=w444) -> ()  [unwired: 6 in, 3 out]
        }
      }
    }
  }
